vi "wrapper_path.vi"(8 "error in (no error)":errorcluster) -> (0 "error out":errorcluster, 3 "wrapper path":path)   [LabVIEW 2017, in "libonnx_wrapper.lvlib"]
uses:
  libonnx_wrapper.lvlib
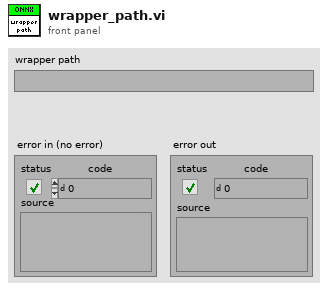
[diagram p1: front panel]
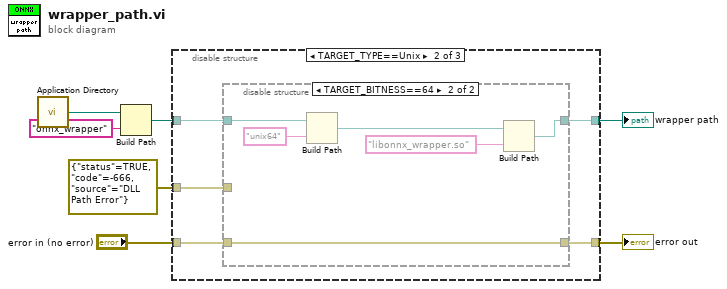
[diagram p0: block diagram]
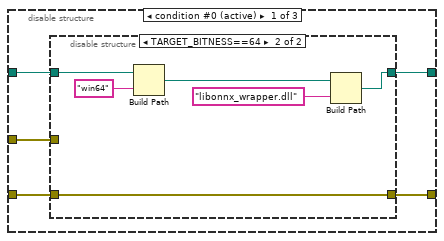
[diagram p2: hidden frame]
diagram:
  n1 = call <vilib>:"Application Directory.vi"() -> ("Application Directory"=w7:path)
  n2 = Build Path(base path=w7, name or relative path="onnx_wrapper") -> (appended path=w3:path)
  n3 = disable-structure shown="TARGET_TYPE==Unix" {
    disable-tunnel: "error in (no error)" -> [w8 w25 _]
    disable-tunnel: [w11 w24 w34] -> w4
    disable-tunnel: w3 -> [w12 w23 _]
    disable-tunnel: [w9 w22 _] -> w2
    disable-tunnel: errorcluster {"status"=TRUE, "code"=-666, "source"="DLL Path Error"} ("error IO") -> [w10 w21 w34]
    frame condition #0 (active) {
      n4 = disable-structure shown="TARGET_BITNESS==64" {
        disable-tunnel: w8 -> [_ w20]
        disable-tunnel: [w13 w20] -> w11
        disable-tunnel: w12 -> [w14 w19]
        disable-tunnel: [w14 w15] -> w9
        disable-tunnel: w10 -> [w13 _]
        frame condition #0 {
        }
        frame condition #1 (active) {
          n5 = Build Path(base path=w19, name or relative path="win64") -> (appended path=w16:path)
          n6 = Build Path(base path=w16, name or relative path="libonnx_wrapper.dll") -> (appended path=w15:path)
        }
      }
    }
    frame condition #1 {
      n7 = disable-structure shown="TARGET_BITNESS==64" {
        disable-tunnel: w25 -> [_ w33]
        disable-tunnel: [w26 w33] -> w24
        disable-tunnel: w23 -> [w27 w32]
        disable-tunnel: [w27 w28] -> w22
        disable-tunnel: w21 -> [w26 _]
        frame condition #0 {
        }
        frame condition #1 (active) {
          n8 = Build Path(base path=w32, name or relative path="unix64") -> (appended path=w29:path)
          n9 = Build Path(base path=w29, name or relative path="libonnx_wrapper.so") -> (appended path=w28:path)
        }
      }
    }
    frame condition #2 {
    }
  }
  "error out" <- w4
  "wrapper path" <- w2
